vi "S2C_5190CR_Proc_TcpOpen.vi"(8 "Error In":errorcluster, 11 "Settings In":T1) -> (0 "Error Out":errorcluster, 2 "TCP_Ref":refnum<k5>, 3 "Settings Out":T1)   [LabVIEW 2015]
doc: "Opens a TCP connection to the given IP address and port."
uses:
  S2C_5190CR_Proc_Globals.vi
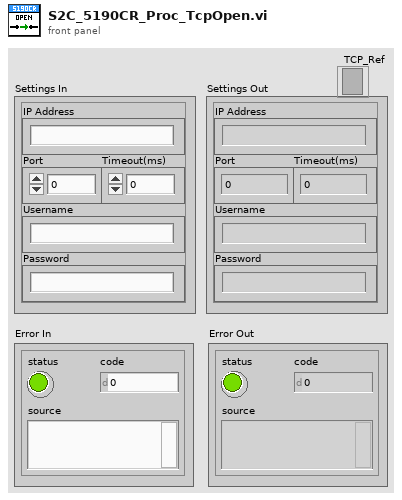
[diagram p1: front panel]
types:
  T1 = cluster{"IP Address":string, "Port":u16, "Username":string, "Password":string, "Timeout(ms)":i32}
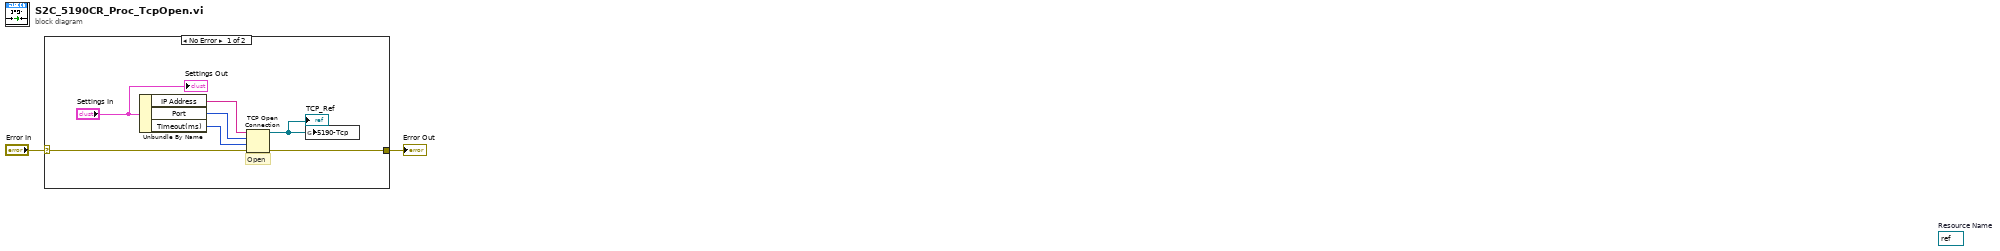
[diagram p0: block diagram]
diagram:
  (unwired) refnum<visa-resource-name> refnum  # Resource Name
  n1 = case shown="No Error" "Error In" {
    selector: "Error In" -> [w9 w10]
    tunnel: [w8 w10] -> w1
    frame No Error {
      # "Open"
      n2 = Unbundle By Name("Settings In") -> ("IP Address"=w5:string, "Port"=w6:u16, "Timeout(ms)"=w7:i32)
      n3 = TCP Open Connection(address=w5, remote port or service name=w6, timeout ms (60000)=w7, error in (no error)=w9) -> (connection ID=w3:refnum<k5>, error out=w8:errorcluster)  [unwired: 1 in]
      "TCP_Ref" <- w3
      n4 = global write "S2C_5190CR_Proc_Globals.vi" "5190-Tcp"(w3) -> ()
      "Settings Out" <- "Settings In"
    }
    frame Error {
    }
  }
  "Error Out" <- w1
